vi "EvaluateGuess.vi"(8 "error in (no error)":errorcluster, 10 "Guess":string, 11 "Controller in":refnum<class "Controller.lvclass">) -> (0 "error out":errorcluster, 1 "correct?":bool, 2 "Result":u32[](array[colorbox]), 3 "Controller out":refnum<class "Controller.lvclass">)   [LabVIEW 2024, in "GUI.lvlib" / "Controller.lvclass"]
uses:
  Controller.lvclass
  Controller.lvclass/Controller.ctl
  TypeDefs/Yellow.ctl
  TypeDefs/Green.ctl
  TypeDefs/Grey.ctl
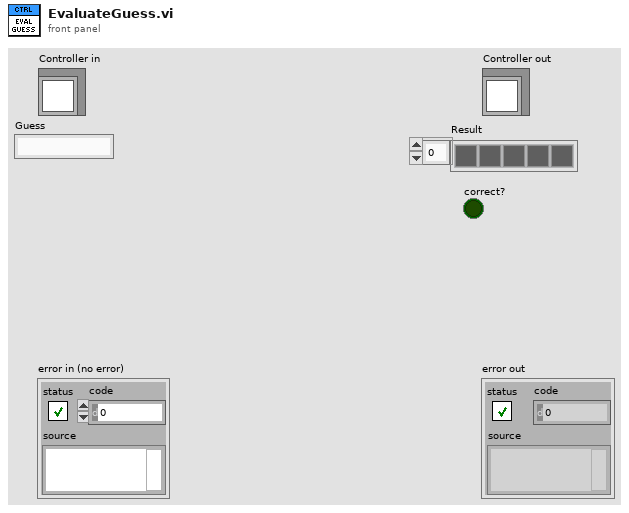
[diagram p1: front panel]
types:
  T1 = typedef "Grey.ctl" = u32
  T2 = typedef "Green.ctl" = u32
  T3 = typedef "Yellow.ctl" = u32
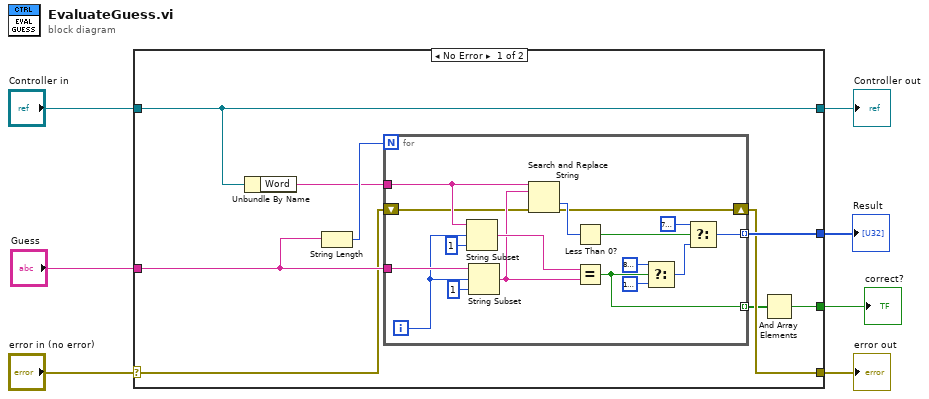
[diagram p0: block diagram]
diagram:
  n1 = case shown="No Error" "error in (no error)" {
    selector: "error in (no error)" -> [w11 w35]
    tunnel: [w10 w35] -> w6
    tunnel: [w16 w34] -> w4
    tunnel: "Controller in" -> [w16 w34]
    tunnel: "Guess" -> [w15 _]
    tunnel: [w13 _] -> w2
    tunnel: [w8 _] -> w1
    frame No Error {
      n2 = Unbundle By Name(w16) -> ("Word"=w12:string)
      n3 = String Length(string=w15) -> (length=w14:i32)
      n4 = for {
        N: w14 -> [_]
        tunnel: w15 -> [w33]
        tunnel: w12 -> [w26]
        tunnel: [w28] -> w13 mode=indexing
        shift-right: [w23] -> w10
        shift-left: w11 -> [w22]
        tunnel: [w20] -> w9 mode=indexing
        i -> [w21]
        n5 = String Subset(string=w26, offset (0)=w21, length (rest)=1 ("length (rest)")) -> (substring=w25:string)
        n6 = String Subset(string=w33, offset (0)=w21, length (rest)=1 ("length (rest)")) -> (substring=w24:string)
        n7 = Search and Replace String(input string=w26, search string=w24, error in=w22) -> (offset past replacement=w30:i32, error out=w23:errorcluster)  [unwired: 5 in, 2 out]
        n8 = Less Than 0?(x=w30) -> (x < 0?=w31:bool)
        n9 = Equal?(x=w25, y=w24) -> (x = y?=w20:bool)
        n10 = Select(t=T2 8173175 ("Green"), s=w20, f=T3 14400581 ("Yellow")) -> (s? t:f=w29:T3)
        n11 = Select(t=T1 7896190 ("Grey"), s=w31, f=w29) -> (s? t:f=w28:T3)
      }
      n12 = And Array Elements(Boolean array=w9) -> (logical AND=w8:bool)
    }
    frame Error {
    }
  }
  "error out" <- w6
  "Controller out" <- w4
  "Result" <- w2
  "correct?" <- w1
